vi "Read XYR.vi"(0 "Lockin SR830 in":refnum<class "Lockin SR830.lvclass">, 11 "error in (no error)":errorcluster) -> (4 "Lockin SR830 out":refnum<class "Lockin SR830.lvclass">, 6 "X":dbl, 8 "Y":dbl, 10 "R":dbl, 15 "error out":errorcluster)   [LabVIEW 2012, in "Lockin SR830.lvclass"]
uses:
  Lockin SR830.lvclass
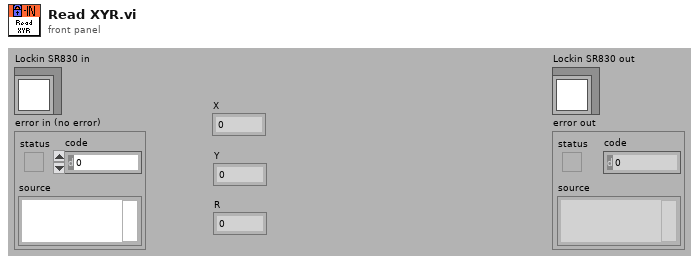
[diagram p1: front panel]
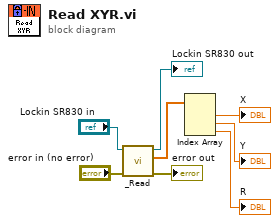
[diagram p0: block diagram]
diagram:
  n1 = call-dynamic "_Read.vi"("error in (no error)"="error in (no error)", "Lockin SR830 in"="Lockin SR830 in") -> ("error out"=→"error out":errorcluster, "4 Data Points"=w4:dbl[], "Lockin SR830 out"=→"Lockin SR830 out":refnum<class "Lockin SR830.lvclass">)  [unwired: 7 in]
  n2 = Index Array(array=w4) -> (element #1=→"X":dbl, element #2=→"Y":dbl, element #3=→"R":dbl)  [unwired: 3 in]
